vi "async_get_start.vi"(8 "error in (no error)":errorcluster, 10 "url":string, 11 "Client in":refnum<class "Client.lvclass">) -> (0 "error out":errorcluster, 2 "Request":refnum<class "Request.lvclass">, 3 "Client out":refnum<class "Client.lvclass">)   [LabVIEW 2020, in "reqwest.lvlib" / "Client.lvclass"]
uses:
  Client.lvclass
  Request/Request.lvclass
  Client.lvclass/Client.ctl
  lv_src/lv_reqwest_64.dll
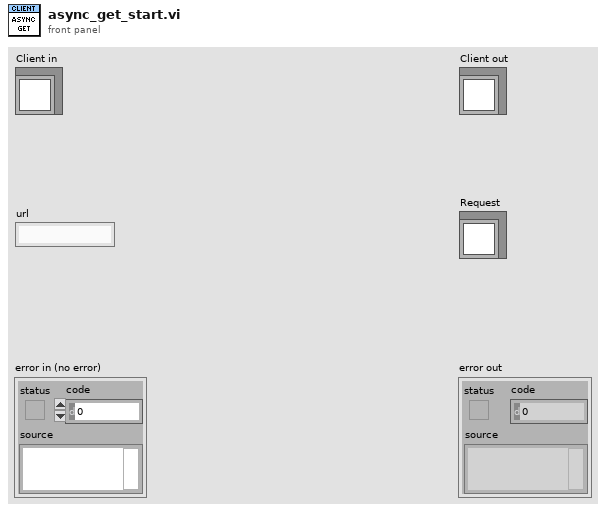
[diagram p1: front panel]
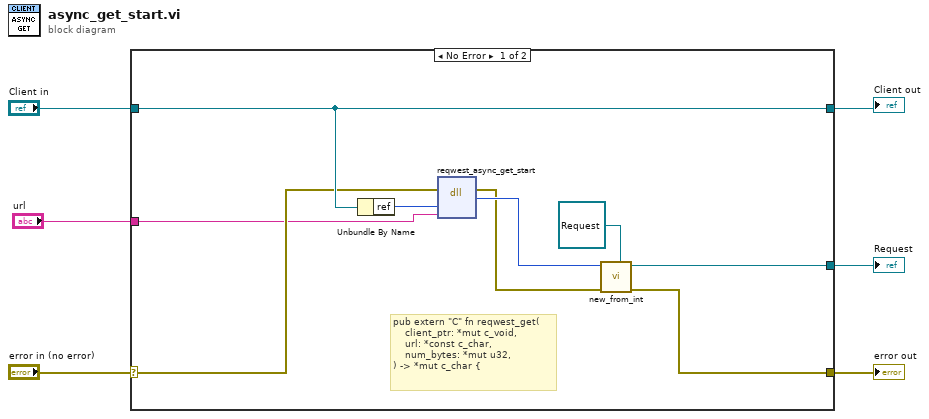
[diagram p0: block diagram]
diagram:
  n1 = case shown="No Error" "error in (no error)" {
    selector: "error in (no error)" -> [w10 w16]
    tunnel: "Client in" -> [w11 w17]
    tunnel: [w12 _] -> w4
    tunnel: [w9 w16] -> w2
    tunnel: [w11 w17] -> w3
    tunnel: "url" -> [w8 _]
    frame No Error {
      # "pub extern \"C\" fn reqwest_get(\n    client_ptr: *mut c_void,\n    url: *const c_char,\n    num_bytes: *mut u32,\n) -> *mut c_char {"
      n2 = Unbundle By Name(w11) -> ("ref"=w13:u64)
      n3 = dll-call lib="C:/Projects/toml-edit-labview/lv_src/lv_reqwest_64.dll" fn="reqwest_async_get_start"(error in=w10, "client_ref"=w13, "url"=w8) -> (error out=w14:errorcluster, "request_id"=w15:i32)  [unwired: 4 in, 1 out]
      n4 = call "new_from_int.vi"("Request in"=refnum<class "Request.lvclass"> refnum, "error in (no error)"=w14, "request_id"=w15) -> ("error out"=w9:errorcluster, "Request out"=w12:refnum<class "Request.lvclass">)  [unwired: 7 in]
    }
    frame Error {
    }
  }
  "error out" <- w2
  "Request" <- w4
  "Client out" <- w3
